vi "command_line_gen.vi"(8 "Use default values":bool, 9 "error in (no error)":errorcluster, 10 "Path":path, 11 "Input parameters":T1) -> (2 "error out":errorcluster, 3 "Command":string)   [LabVIEW 2019]
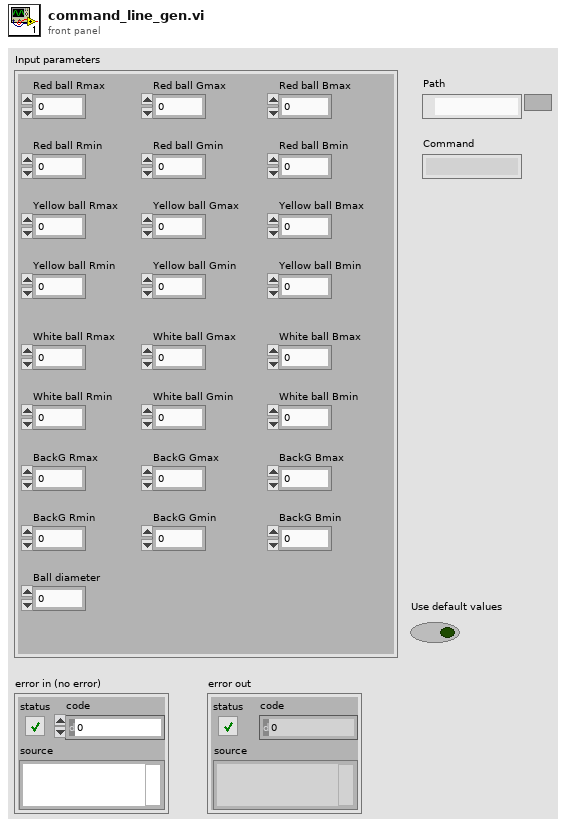
[diagram p1: front panel]
types:
  T1 = cluster{"Red ball Rmax":u8, "Red ball Gmax":u8, "Red ball Bmax":u8, "Red ball Rmin":u8, "Red ball Gmin":u8, "Red ball Bmin":u8, "Yellow ball Rmax":u8, "Yellow ball Gmax":u8, "Yellow ball Bmax":u8, "Yellow ball Rmin":u8, "Yellow ball Gmin":u8, "Yellow ball Bmin":u8, "White ball Rmax":u8, "White ball Gmax":u8, "White ball Bmax":u8, "White ball Rmin":u8, "White ball Gmin":u8, "White ball Bmin":u8, "BackG Rmax":u8, "BackG Gmax":u8, "BackG Bmax":u8, "BackG Rmin":u8, "BackG Gmin":u8, "BackG Bmin":u8, "Ball diameter":u8}
  T2 = cluster{"R max":u8, "R min":u8, "G max":u8, "G min":u8, "B max":u8, "B min":u8}
  T3 = cluster{"left":i32, "top":i32, "right":i32, "bottom":i32}
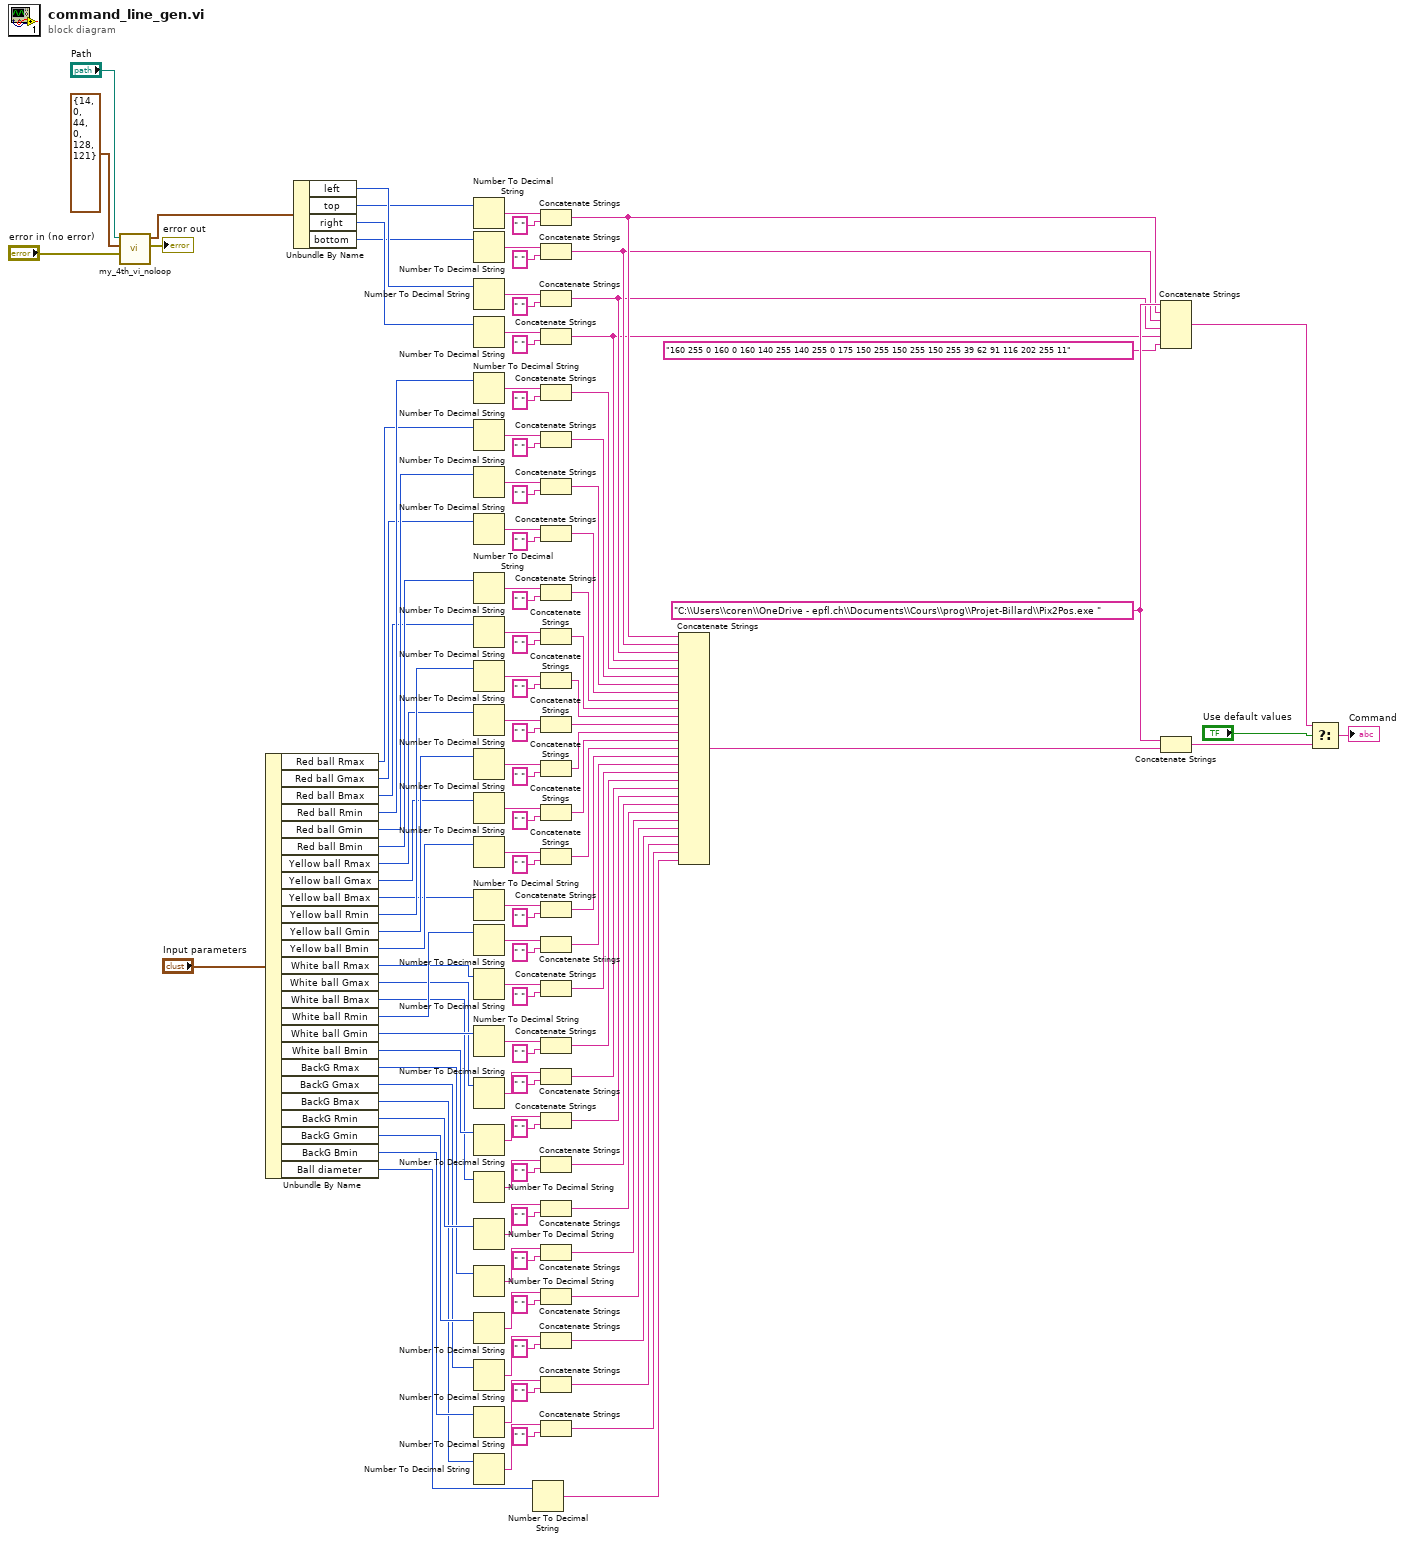
[diagram p0: block diagram]
diagram:
  w7 = "C:\\Users\\coren\\OneDrive - epfl.ch\\Documents\\Cours\\prog\\Projet-Billard\\Pix2Pos.exe " ("string")
  n1 = call "my_4th_vi_noloop.vi"("error in (no error)"="error in (no error)", "Color range"=T2 {"R max"=14, "R min"=0, "G max"=44, "G min"=0, "B max"=128, "B min"=121}, "PNG file"="Path") -> ("error out"=→"error out":errorcluster, "Billard rect"=w123:T3)  [unwired: 7 in]
  n2 = Unbundle By Name("Input parameters") -> ("Red ball Rmax"=w103:u8, "Red ball Gmax"=w95:u8, "Red ball Bmax"=w87:u8, "Red ball Rmin"=w107:u8, "Red ball Gmin"=w99:u8, "Red ball Bmin"=w91:u8, "Yellow ball Rmax"=w71:u8, "Yellow ball Gmax"=w67:u8, "Yellow ball Bmax"=w63:u8, "Yellow ball Rmin"=w73:u8, "Yellow ball Gmin"=w69:u8, "Yellow ball Bmin"=w65:u8, "White ball Rmax"=w47:u8, "White ball Gmax"=w43:u8, "White ball Bmax"=w39:u8, "White ball Rmin"=w49:u8, "White ball Gmin"=w45:u8, "White ball Bmin"=w41:u8, "BackG Rmax"=w23:u8, "BackG Gmax"=w19:u8, "BackG Bmax"=w15:u8, "BackG Rmin"=w25:u8, "BackG Gmin"=w21:u8, "BackG Bmin"=w17:u8, "Ball diameter"=w13:u8)
  n3 = Unbundle By Name(w123) -> ("left"=w122:i32, "top"=w120:i32, "right"=w118:i32, "bottom"=w116:i32)
  n4 = Number To Decimal String(number=w120) -> (decimal integer string=w119:string)  [unwired: 1 in]
  n5 = Number To Decimal String(number=w116) -> (decimal integer string=w115:string)  [unwired: 1 in]
  n6 = Number To Decimal String(number=w122) -> (decimal integer string=w121:string)  [unwired: 1 in]
  n7 = Number To Decimal String(number=w118) -> (decimal integer string=w117:string)  [unwired: 1 in]
  n8 = Number To Decimal String(number=w107) -> (decimal integer string=w109:string)  [unwired: 1 in]
  n9 = Number To Decimal String(number=w103) -> (decimal integer string=w105:string)  [unwired: 1 in]
  n10 = Number To Decimal String(number=w99) -> (decimal integer string=w101:string)  [unwired: 1 in]
  n11 = Number To Decimal String(number=w95) -> (decimal integer string=w97:string)  [unwired: 1 in]
  n12 = Number To Decimal String(number=w91) -> (decimal integer string=w93:string)  [unwired: 1 in]
  n13 = Number To Decimal String(number=w87) -> (decimal integer string=w89:string)  [unwired: 1 in]
  n14 = Number To Decimal String(number=w73) -> (decimal integer string=w85:string)  [unwired: 1 in]
  n15 = Number To Decimal String(number=w71) -> (decimal integer string=w83:string)  [unwired: 1 in]
  n16 = Number To Decimal String(number=w69) -> (decimal integer string=w81:string)  [unwired: 1 in]
  n17 = Number To Decimal String(number=w67) -> (decimal integer string=w79:string)  [unwired: 1 in]
  n18 = Number To Decimal String(number=w65) -> (decimal integer string=w77:string)  [unwired: 1 in]
  n19 = Number To Decimal String(number=w63) -> (decimal integer string=w75:string)  [unwired: 1 in]
  n20 = Number To Decimal String(number=w49) -> (decimal integer string=w61:string)  [unwired: 1 in]
  n21 = Number To Decimal String(number=w47) -> (decimal integer string=w59:string)  [unwired: 1 in]
  n22 = Number To Decimal String(number=w45) -> (decimal integer string=w57:string)  [unwired: 1 in]
  n23 = Number To Decimal String(number=w43) -> (decimal integer string=w55:string)  [unwired: 1 in]
  n24 = Number To Decimal String(number=w41) -> (decimal integer string=w53:string)  [unwired: 1 in]
  n25 = Number To Decimal String(number=w39) -> (decimal integer string=w51:string)  [unwired: 1 in]
  n26 = Number To Decimal String(number=w25) -> (decimal integer string=w27:string)  [unwired: 1 in]
  n27 = Number To Decimal String(number=w23) -> (decimal integer string=w37:string)  [unwired: 1 in]
  n28 = Number To Decimal String(number=w21) -> (decimal integer string=w35:string)  [unwired: 1 in]
  n29 = Number To Decimal String(number=w19) -> (decimal integer string=w33:string)  [unwired: 1 in]
  n30 = Number To Decimal String(number=w17) -> (decimal integer string=w31:string)  [unwired: 1 in]
  n31 = Number To Decimal String(number=w15) -> (decimal integer string=w29:string)  [unwired: 1 in]
  n32 = Number To Decimal String(number=w13) -> (decimal integer string=w11:string)  [unwired: 1 in]
  n33 = Concatenate Strings(w119, " " ("string")) -> (w6:string)
  n34 = Concatenate Strings(w115, " " ("string")) -> (w5:string)
  n35 = Concatenate Strings(w121, " " ("string")) -> (w4:string)
  n36 = Concatenate Strings(w117, " " ("string")) -> (w3:string)
  n37 = Concatenate Strings(w109, " " ("string")) -> (w106:string)
  n38 = Concatenate Strings(w105, " " ("string")) -> (w102:string)
  n39 = Concatenate Strings(w101, " " ("string")) -> (w98:string)
  n40 = Concatenate Strings(w97, " " ("string")) -> (w94:string)
  n41 = Concatenate Strings(w93, " " ("string")) -> (w90:string)
  n42 = Concatenate Strings(w89, " " ("string")) -> (w86:string)
  n43 = Concatenate Strings(w85, " " ("string")) -> (w72:string)
  n44 = Concatenate Strings(w83, " " ("string")) -> (w70:string)
  n45 = Concatenate Strings(w81, " " ("string")) -> (w68:string)
  n46 = Concatenate Strings(w79, " " ("string")) -> (w66:string)
  n47 = Concatenate Strings(w77, " " ("string")) -> (w64:string)
  n48 = Concatenate Strings(w75, " " ("string")) -> (w62:string)
  n49 = Concatenate Strings(w61, " " ("string")) -> (w48:string)
  n50 = Concatenate Strings(w59, " " ("string")) -> (w46:string)
  n51 = Concatenate Strings(w57, " " ("string")) -> (w44:string)
  n52 = Concatenate Strings(w55, " " ("string")) -> (w42:string)
  n53 = Concatenate Strings(w53, " " ("string")) -> (w40:string)
  n54 = Concatenate Strings(w51, " " ("string")) -> (w38:string)
  n55 = Concatenate Strings(w27, " " ("string")) -> (w24:string)
  n56 = Concatenate Strings(w37, " " ("string")) -> (w22:string)
  n57 = Concatenate Strings(w35, " " ("string")) -> (w20:string)
  n58 = Concatenate Strings(w33, " " ("string")) -> (w18:string)
  n59 = Concatenate Strings(w31, " " ("string")) -> (w16:string)
  n60 = Concatenate Strings(w29, " " ("string")) -> (w14:string)
  n61 = Concatenate Strings(w6, w5, w4, w3, w106, w102, w98, w94, w90, w86, w72, w70, w68, w66, w64, w62, w48, w46, w44, w42, w40, w38, w24, w22, w20, w18, w16, w14, w11) -> (w12:string)
  n62 = Concatenate Strings(w7, w6, w5, w4, w3, "160 255 0 160 0 160 140 255 140 255 0 175 150 255 150 255 150 255 39 62 91 116 202 255 11" ("string")) -> (w1:string)
  n63 = Concatenate Strings(w7, w12) -> (w9:string)
  n64 = Select(t=w1, s="Use default values", f=w9) -> (s? t:f=→"Command":string)
